vi "策略设计设计模式DEMO.vi"() -> ()   [LabVIEW 2013]
uses:
  Strategy_class/Operation Context.lvclass
  <vilib>/addons/_AddQ/G#Object/G#Object.lvclass
  Add_class/Add.lvclass
  Mul_class/Mul.lvclass
panel:
  in  "停止":bool
  out "# of objects killed":i32
  out "Output":string
  out "result":dbl
  in  "y":dbl
  in  "x":dbl
  in  "Operation":enum16{"Add", "Mul"}(ring)
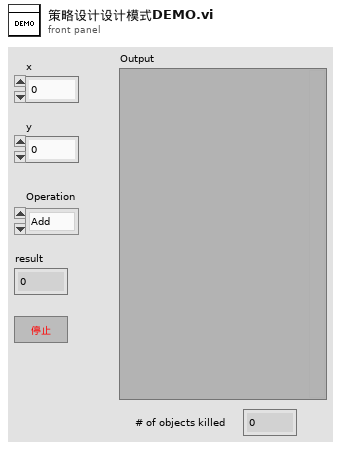
[diagram p1: front panel]
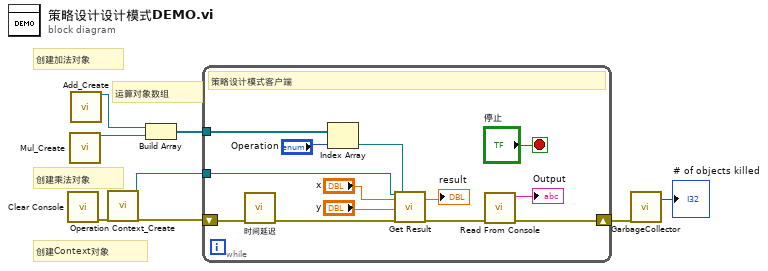
[diagram p0: block diagram]
diagram:
  # "运算对象数组"
  # "创建乘法对象"
  # "创建Context对象"
  # "创建加法对象"
  n1 = call "Clear Console.vi"() -> ("error out"=w6:errorcluster)  [unwired: 11 in]
  n2 = call "Mul_Create.vi"() -> ("reference out"=w2:refnum<class "Mul.lvclass">)  [unwired: 18 in, 1 out]
  n3 = call "Add_Create.vi"() -> ("reference out"=w3:refnum<class "Add.lvclass">)  [unwired: 18 in, 1 out]
  n4 = call "Operation Context_Create.vi"("error in (no error)"=w6) -> ("reference out"=w4:refnum<class "Operation Context.lvclass">, "error out"=w5:errorcluster)  [unwired: 17 in]
  n5 = Build Array(w3, w2) -> (w1:refnum<class "Operation.lvclass">[])
  n6 = while {
    shift-right: [w20] -> w8
    shift-left: w5 -> [w21]
    tunnel: w4 -> [w9]
    tunnel: w1 -> [w12]
    stop <- "停止" stop-if-true
    # "策略设计模式客户端"
    n7 = call "时间延迟"("error in (no error)"=w21) -> ("error out"=w17:errorcluster)  [unwired: 10 in]
    n8 = Index Array(array=w12, index="Operation") -> (element=w10:refnum<class "Operation.lvclass">)
    n9 = call-dynamic "Get Result.vi"("reference in"=w9, "x"="x", "y"="y", "error in (no error)"=w17, "Operation.lvclass"=w10) -> ("result"=→"result":dbl, "error out"=w13:errorcluster)  [unwired: 12 in, 1 out]
    n10 = call "Read From Console.vi"("error in (no error)"=w13) -> ("error out"=w20:errorcluster, "Output"=→"Output":string)  [unwired: 9 in]
  }
  n11 = call <vilib>:"GarbageCollector.vi"("error in (no error)"=w8) -> ("# of objects killed"=→"# of objects killed":i32)  [unwired: 16 in, 2 out]
